vi "He3 Mano Read.vi"(2 "Range":i32(ring)=2 items=["range X0.01", "range X0.1", "range X1"], 3 "GPIB Address":string="15") -> (0 "3He Temp (K)":dbl format="%.3f", 1 "3He Pressure (Torr)":dbl format="%.3f")   [LabVIEW 2009]
doc: "This VI reads the MKS 270 at the given gpib address and returns both the 3He pressure and corresponding temperature, in Kelvin."
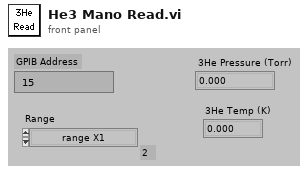
[diagram p1: front panel]
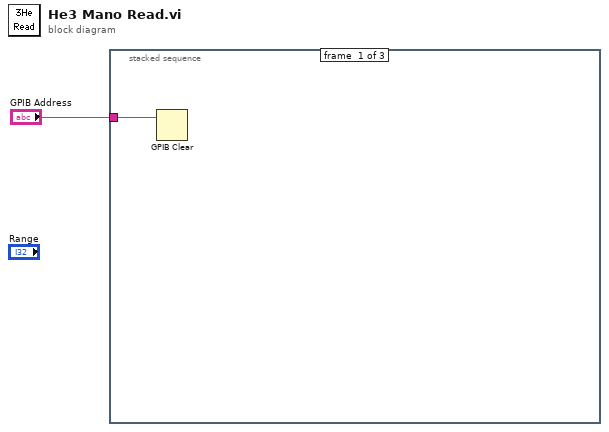
[diagram p0: block diagram]
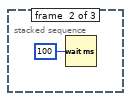
[diagram p2: hidden frame]
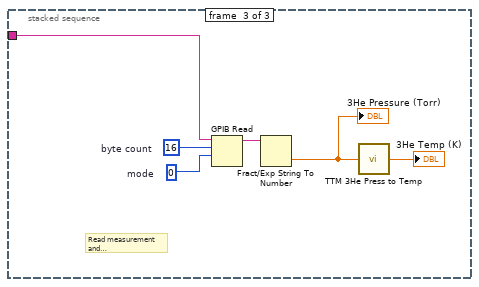
[diagram p3: hidden frame]
diagram:
  n1 = stacked-sequence {
    tunnel: "GPIB Address" -> [w2 _ w5]
    frame #0 {
      n2 = GPIB Clear(3:w2) -> ()  [unwired: 1 in, 2 out]
    }
    frame #1 {
      n3 = Wait (ms)(milliseconds to wait=u32 100) -> ()  [unwired: 1 out]
    }
    frame #2 {
      w8 = 16  # byte count
      w9 = 0  # mode
      # "Read measurement and \nconvert it to numeric"
      n4 = GPIB Read(0:w5, 1:w8, 2:w9) -> (5:w7:string)  [unwired: 2 in, 2 out]
      n5 = Fract/Exp String To Number(string=w7) -> (number=w4:dbl)  [unwired: 3 in, 1 out]
      "3He Pressure (Torr)" <- w4
      n6 = call "TTM 3He Press to Temp.vi"("3He Vapor pressure in mmhg  between  0.02 and 200."=w4) -> ("corresponding temp K"=→"3He Temp (K)":dbl)
    }
  }
